vi "Read 32-bit first word low.vi"(8 "error in (no error)":errorcluster, 11 "Modbus Module configuration in":refnum<class "Modbus Module configuration.lvclass">) -> (0 "error out":errorcluster, 2 "32-bit: first word low":bool, 3 "Modbus Module configuration out":refnum<class "Modbus Module configuration.lvclass">)   [LabVIEW 2014, in "Modbus Module configuration.lvclass"]
uses:
  Modbus Module configuration.lvclass
  Modbus Module configuration.lvclass/Modbus Module configuration.ctl
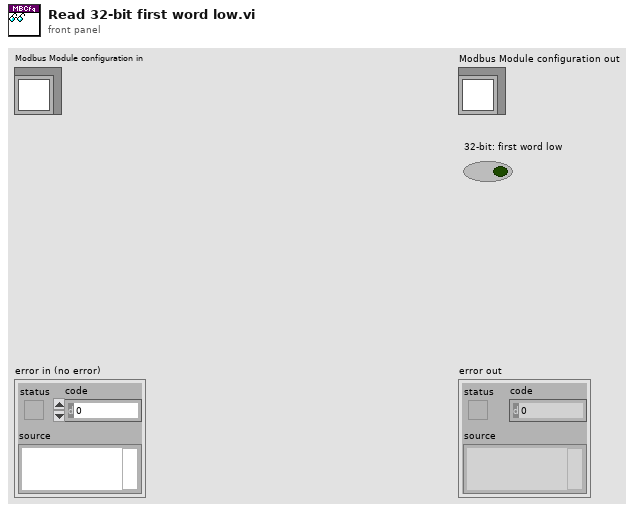
[diagram p1: front panel]
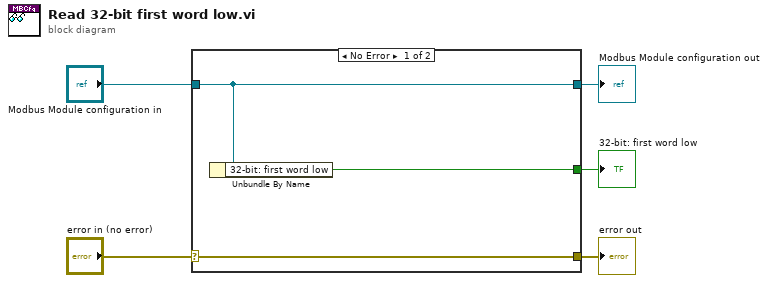
[diagram p0: block diagram]
diagram:
  n1 = case shown="No Error" "error in (no error)" {
    selector: "error in (no error)" -> [w8 w9]
    tunnel: [w8 w9] -> w4
    tunnel: [w7 w10] -> w2
    tunnel: "Modbus Module configuration in" -> [w7 w10]
    tunnel: [w6 _] -> w1
    frame No Error {
      n2 = Unbundle By Name(w7) -> ("32-bit: first word low"=w6:bool)
    }
    frame Error {
    }
  }
  "error out" <- w4
  "Modbus Module configuration out" <- w2
  "32-bit: first word low" <- w1
